vi "Find all vis with no caller.vi"() -> ()   [LabVIEW 2013]
doc: "Finds all .vis in the project that have no callers. These .vis can be opened using this vi."
panel:
  out "name":string
  out "progress":i32(slide) scale=0.0..1157.0
  in  "State":T1(ring)=enum."Minimized"
  in  "Open F.Ps?":bool
  out "size(s)":i32
  out "Array":cluster{"stripped path":path, "name":string}[](array[cluster])
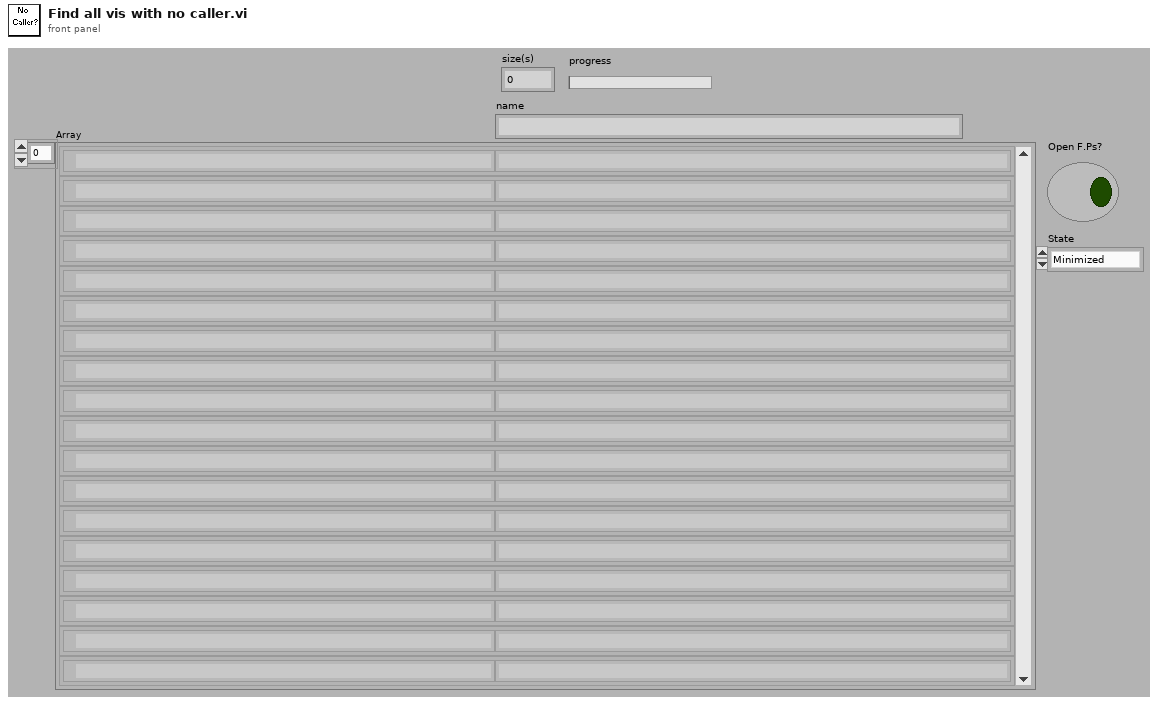
[diagram p1: front panel]
types:
  T1 = enum32{"Invalid", "Standard", "Closed", "Hidden", "Minimized", "Maximized"}
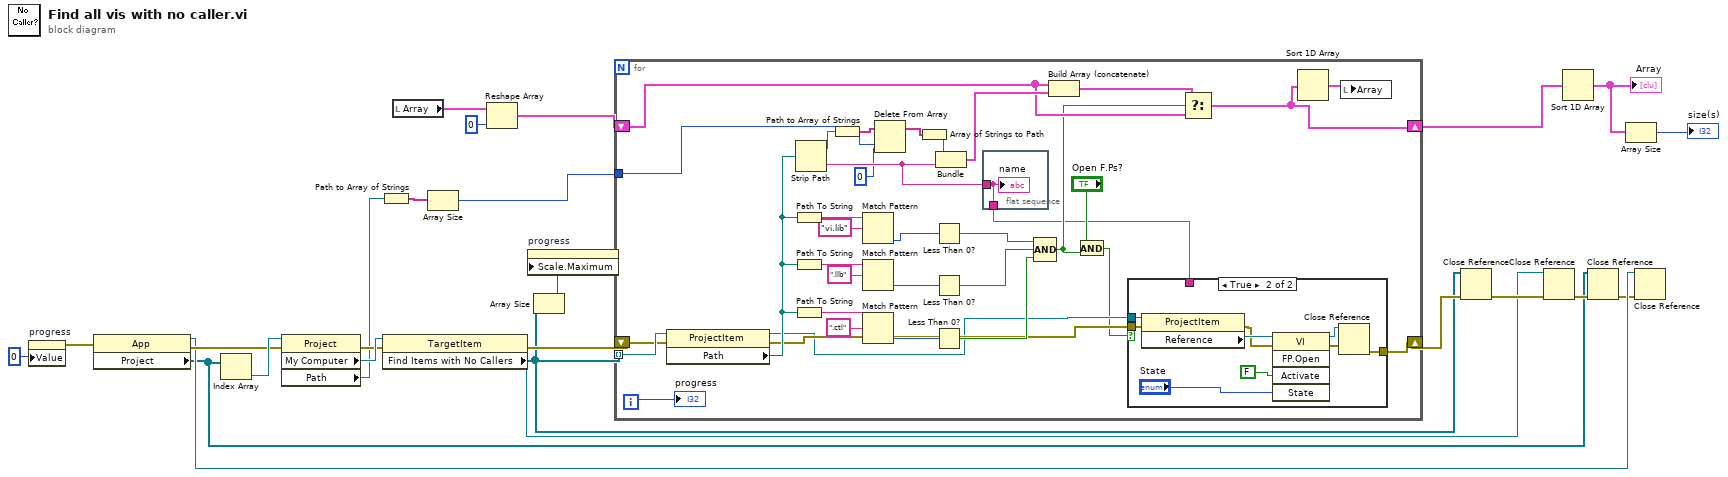
[diagram p0: block diagram]
diagram:
  n1 = property on="progress" class="Slide (strict)"("Value"=0 ("progress")) -> (error out=w4:errorcluster)  [unwired: 2 in, 1 out]
  n2 = property class="App"(error in=w4) -> (reference out=w16:refnum<vi>, error out=w18:errorcluster, "Project"=w8:refnum<vi>[])  [unwired: 1 in]
  n3 = Index Array(array=w8) -> (element=w21:refnum<vi>)  [unwired: 1 in]
  n4 = property class="Project"(reference=w21, error in=w18) -> (error out=w19:errorcluster, "My Computer"=w25:refnum<vi>, "Path"=w3:path)  [unwired: 1 out]
  n5 = Path to Array of Strings(0:w3) -> (2:w2:string[])  [unwired: 1 out]
  n6 = property class="TargetItem"(reference=w25, error in=w19) -> (reference out=w11:refnum<vi>, error out=w20:errorcluster, "Find Items with No Callers"=w7:refnum<vi>[])
  n7 = local read "Array"() -> (w15:cluster{"stripped path":path, "name":string}[])
  n8 = Array Size(array=w2) -> (size(s)=w1:i32)
  n9 = Reshape Array(w15, 0 ("dimension size")) -> (w14:cluster{"stripped path":path, "name":string}[])
  n10 = Array Size(array=w7) -> (size(s)=w6:i32)
  n11 = property on="progress" class="Slide (strict)"("Scale.Maximum"=w6) -> ()  [unwired: 2 in, 2 out]
  n12 = for {
    tunnel: w7 -> [w60] mode=indexing
    shift-right: [w28] -> w24
    shift-left: w14 -> [w47]
    shift-right: [w32] -> w17
    shift-left: w20 -> [w55]
    tunnel: w1 -> [w26]
    i -> [w30]
    n13 = property class="ProjectItem"(reference=w60, error in=w55) -> (reference out=w35:refnum<vi>, error out=w36:errorcluster, "Path"=w38:path)
    n14 = Path To String(path=w38) -> (string=w59:string)
    n15 = Path To String(path=w38) -> (string=w45:string)
    n16 = Path To String(path=w38) -> (string=w40:string)
    n17 = Strip Path(path=w38) -> (stripped path=w52:path, name=w54:string)
    n18 = Path to Array of Strings(0:w52) -> (2:w51:string[])  [unwired: 1 out]
    n19 = Match Pattern(string=w59, regular expression="vi.lib") -> (offset past match=w57:i32)  [unwired: 4 out]
    n20 = Match Pattern(string=w45, regular expression=".llb") -> (offset past match=w44:i32)  [unwired: 4 out]
    n21 = Match Pattern(string=w40, regular expression=".ctl") -> (offset past match=w41:i32)  [unwired: 4 out]
    n22 = Delete From Array(array=w51, length=w26, index=0) -> (array with subset deleted=w50:string[])  [unwired: 1 out]
    n23 = Array of Strings to Path(0:w50) -> (2:w49:path)  [unwired: 1 out]
    n24 = Less Than 0?(x=w57) -> (x < 0?=w43:bool)
    n25 = Less Than 0?(x=w44) -> (x < 0?=w42:bool)
    n26 = Less Than 0?(x=w41) -> (x < 0?=w37:bool)
    n27 = Bundle("path"=w49, "name"=w54) -> (w53:cluster{"path":path, "name":string})  [unwired: 1 out]
    n28 = flat-sequence {
      tunnel: w54 -> [w61]
      tunnel: [w61] -> w27
      frame #0 {
        "name" <- w61
      }
    }
    n29 = Compound Arithmetic op=AND(w43, w42, w37) -> (w33:bool)
    n30 = Build Array (concatenate)(w47, w53) -> (w56:cluster{"path":path, "name":string}[])
    n31 = And(x="Open F.Ps?", y=w33) -> (x .and. y?=w31:bool)
    n32 = case shown="True" w31 {
      tunnel: w36 -> [w62 w71]
      tunnel: w35 -> [_ w70]
      tunnel: [w62 w64] -> w32
      tunnel: w27 -> [_ _]
      frame False {
      }
      frame True {
        n33 = property class="ProjectItem"(reference=w70, error in=w71) -> (error out=w63:errorcluster, "Reference"=w69:refnum<vi>)  [unwired: 1 out]
        n34 = invoke class="VI" method="FP.Open"(reference=w69, error in=w63, "Activate"=FALSE ("Activate?"), "State"="State") -> (reference out=w65:refnum<vi>, error out=w66:errorcluster)  [unwired: 1 in, 3 out]
        n35 = Close Reference(reference=w65, error in (no error)=w66) -> (error out=w64:errorcluster)
      }
    }
    n36 = Select(t=w56, s=w33, f=w47) -> (s? t:f=w28:cluster{"stripped path":path, "name":string}[])
    n37 = Sort 1D Array(array=w28) -> (sorted array=w29:cluster{"stripped path":path, "name":string}[])
    n38 = local write "Array"(w29) -> ()
    "progress" <- w30
  }
  n39 = Close Reference(reference=w7, error in (no error)=w17) -> (error out=w12:errorcluster)
  n40 = Close Reference(reference=w11, error in (no error)=w12) -> (error out=w10:errorcluster)
  n41 = Sort 1D Array(array=w24) -> (sorted array=w23:cluster{"stripped path":path, "name":string}[])
  "Array" <- w23
  n42 = Close Reference(reference=w8, error in (no error)=w10) -> (error out=w9:errorcluster)
  n43 = Array Size(array=w23) -> (size(s)=→"size(s)":i32)
  n44 = Close Reference(reference=w16, error in (no error)=w9) -> ()  [unwired: 1 out]
